vi "Deep Learning Object Detection - Overlay Results.vi"(6 "base path":path, 7 "Image Scaling":cluster{"X":dbl, "Y":dbl}, 8 "error in (no error)":errorcluster, 9 "Minimum Score Threshold":sgl=0.5, 10 "Detected Objects":T3[](array[typedef]) {"Bounding Box"."y" format="%.2f"; "Bounding Box"."x" format="%.2f"}, 11 "Image In":T2) -> (0 "error out":errorcluster, 1 "Array":string[](array[string]), 3 "Image Out":T2)   [LabVIEW 2023]
uses:
  <vilib>/vision/Deep Learning.llb/IMAQ DL Model Objects.ctl
  <vilib>/vision/Image Controls.llb/IMAQ Image.ctl
  <vilib>/Utility/file.llb/Read Delimited Spreadsheet (string).vi
panel:
  in  "Font":T1={"Desired Font (Application)"=enum."User-specified Font", "[User-specified Font]"={"Font Name"="Segoe UI", "Size"=24, "Strikeout?"=FALSE, "Italic?"=FALSE, "Underline?"=FALSE, "Outline?"=FALSE, "Shadow?"=FALSE, "Bold?"=TRUE, "Rotation Angle"=0.0}, "Horizontal Alignment"=0, "Vertical Alignment"=0} {"Vertical Alignment" items=["Bottom", "Top", "Baseline"]; "Horizontal Alignment" items=["Left", "Center", "Right"]; "[User-specified Font]"."Rotation Angle" format="%.2f"}
  in  "Color Box":u32(colorbox)=16711680
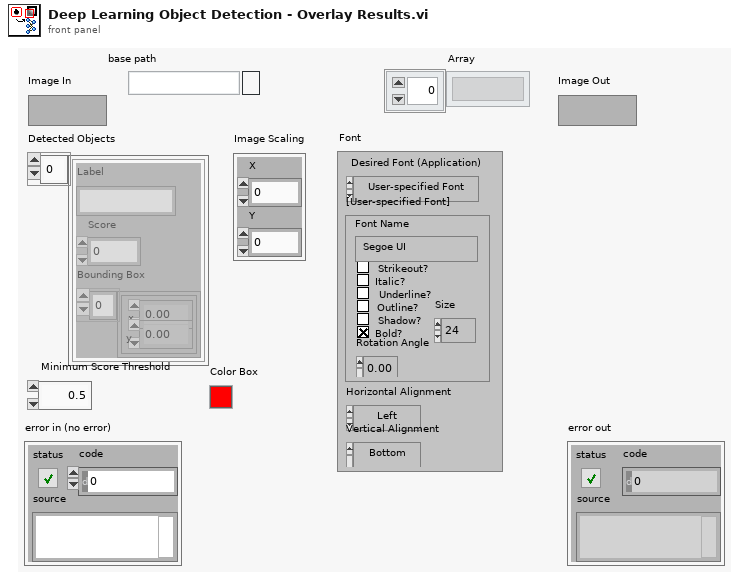
[diagram p1: front panel]
types:
  T1 = cluster{"Desired Font (Application)":enum16{"User-specified Font", "Application Font", "System Font", "Dialog Font"}, "[User-specified Font]":cluster{"Font Name":string, "Size":i16, "Strikeout?":bool, "Italic?":bool, "Underline?":bool, "Outline?":bool, "Shadow?":bool, "Bold?":bool, "Rotation Angle":dbl}, "Horizontal Alignment":i16, "Vertical Alignment":i16}
  T2 = typedef "IMAQ Image.ctl" = refnum<image>
  T3 = typedef "IMAQ DL Model Objects.ctl" = cluster{"Label":string, "Score":sgl, "Bounding Box":cluster{"x":sgl, "y":sgl}[]}
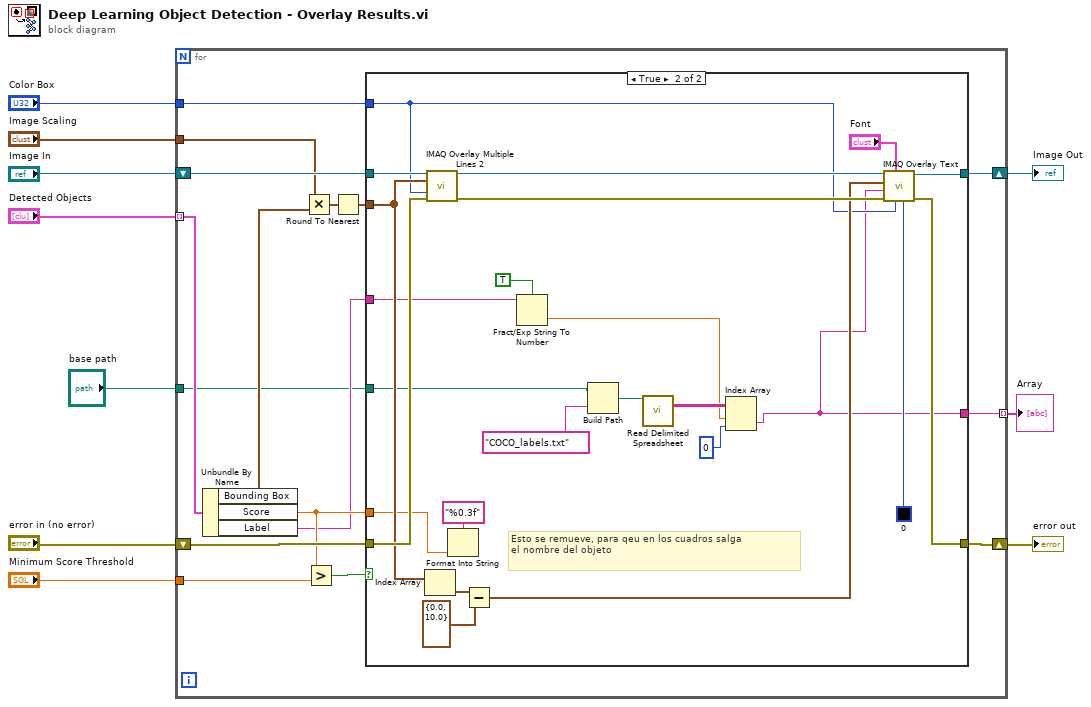
[diagram p0: block diagram]
diagram:
  n1 = for {
    tunnel: "Detected Objects" -> [w26] mode=indexing
    shift-right: [w22] -> w5
    shift-left: "error in (no error)" -> [w23]
    shift-right: [w21] -> w9
    shift-left: "Image In" -> [w25]
    tunnel: "Minimum Score Threshold" -> [w20]
    tunnel: "Color Box" -> [w18]
    tunnel: "Image Scaling" -> [w16]
    tunnel: "base path" -> [w12]
    tunnel: [w11] -> w1 mode=indexing
    n2 = Unbundle By Name(w26) -> ("Bounding Box"=w17:cluster{"x":sgl, "y":sgl}[], "Score"=w19:sgl, "Label"=w13:string)
    n3 = Multiply(x=w16, y=w17) -> (x*y=w15:cluster{dbl, dbl}[])
    n4 = Greater?(x=w19, y=w20) -> (0:w24:bool)
    n5 = Round To Nearest(number=w15) -> (nearest integer value=w14:cluster{dbl, dbl}[])
    n6 = case shown="True" w24 {
      tunnel: w25 -> [w27 w52]
      tunnel: w14 -> [_ w46]
      tunnel: w23 -> [w28 w51]
      tunnel: [w28 w47] -> w22
      tunnel: [w27 w48] -> w21
      tunnel: w19 -> [_ w42]
      tunnel: w18 -> [_ w40]
      tunnel: w13 -> [_ w31]
      tunnel: w12 -> [_ w30]
      tunnel: [_ w29] -> w11
      frame False {
      }
      frame True {
        # "Esto se remueve, para qeu en los cuadros salga\nel nombre del objeto"
        n7 = Index Array(array=w46) -> (element=w45:cluster{dbl, dbl})  [unwired: 1 in]
        n8 = call "IMAQ Overlay Multiple Lines 2"("Image"=w52, "Line End Points"=w46, "Color"=w40, "error in (no error)"=w51) -> ("Image Out"=w50:T2, "error out"=w49:errorcluster)  [unwired: 10 in]
        n9 = Format Into String(format string="%0.3f", w42) -> ()  [unwired: 2 in, 2 out]
        n10 = Subtract(x=w45, y=cluster{"X":dbl, "Y":dbl} {"X"=0.0, "Y"=10.0}) -> (x-y=w43:cluster{dbl, dbl})
        n11 = Fract/Exp String To Number(use system decimal point (T)=TRUE, string=w31) -> (number=w32:dbl)  [unwired: 2 in, 1 out]
        n12 = Build Path(base path=w30, name or relative path="COCO_labels.txt") -> (appended path=w37:path)
        n13 = call-poly <vilib>:"Read Delimited Spreadsheet.vi"("file path (dialog if empty)"=w37) -> ("all rows"=w35:string[][])  [unwired: 9 in, 5 out]
        n14 = Index Array(array=w35, index (row)=w32, index (col)=0 ("index (row)")) -> (element=w29:string)
        n15 = call "IMAQ Overlay Text"("BG Color (Transparent)"=u32 0, "Text Color (black)"=w40, "Font, Size & Style"="Font", "error in (no error)"=w49, "String"=w29, "Origin"=w43, "Image"=w50) -> ("error out"=w47:errorcluster, "Image Out"=w48:T2)  [unwired: 3 in]
      }
    }
  }
  "Image Out" <- w9
  "error out" <- w5
  "Array" <- w1
